vi "TestManyPublications.vi"(8 "error in (no error)":errorcluster, 11 "TestPublishRate In":refnum<class "TestManyPublications.lvclass">) -> (0 "error out":errorcluster, 3 "TestPublishRate Out":refnum<class "TestManyPublications.lvclass">)   [LabVIEW 2017, in "TestManyPublications.lvclass"]
uses:
  TestManyPublications.lvclass
  Source/Framework/IViewModel/IViewModel/IViewModel.lvclass
  C:/Git/mva-framework/Source/Framework/IViewManager/IViewManager/IViewManager.lvclass
  C:/Program Files (x86)/National Instruments/LabVIEW 2017/vi.lib/ActorFramework/Actor/Actor.lvclass
  Source/Framework/IViewable/IViewable/IViewable.lvclass
  Doubles/TestModelManyTopics/TestModelManyTopics.lvclass
  C:/Git/mva-framework/Source/Framework/IModel/IModel/IModel.lvclass
  Source/Framework/Mediator/Mediator/Mediator.lvclass
  C:/Git/mva-framework/Source/Framework/IMediator/IMediator/IMediator.lvclass
  Source/Framework/SubscriptionPolicy/ValueChangeSubscription/ValueChangeSubscription.lvclass/ValueChangeSubscription.ctl
  Source/Framework/IViewModel/IViewModel/IViewModel.lvclass/IViewModel.ctl
  Source/Framework/IViewManager/IViewManager Messages/Launch Nested Views Msg/Launch Nested Views Msg.lvclass/Launch Nested Views Msg.ctl
  Source/Framework/IViewManager/IViewManager/IViewManager.lvclass/IViewManager.ctl
  Source/Framework/Transport/QueueTransport/QueueTransport.lvclass/QueueTransport.ctl
  Source/Framework/IMediator/SubscriptionRequest/SubscriptionRequest.lvclass/SubscriptionRequest.ctl
  Source/Framework/IObserver/IObserver Messages/Subscribe Msg/Subscribe Msg.lvclass/Subscribe Msg.ctl
  <vilib>/ActorFramework/Message Enqueuer/Message Enqueuer.lvclass/Message Enqueuer.ctl
  <vilib>/ActorFramework/Stop Msg/Stop Msg.lvclass/Stop Msg.ctl
  540f04fc-0b85-431b-8f57-02b9bbd5a47e.vi
  81cf93a4-50d8-414a-8355-1077334c3962.vi
  Source/Framework/IViewModel/IViewModel/Write Startup Model-View Configuration.vi
  <vilib>/ActorFramework/Message Enqueuer/Enqueue.vi
  <vilib>/ActorFramework/Message Enqueuer/Enqueue Critical.vi
  Source/Framework/IViewManager/IViewManager Messages/Launch Nested Views Msg/Pack Launch Nested Views Msg.vi
  Source/Framework/IViewManager/IViewManager/Write Startup Launch Nested Views Msg.vi
  Source/Framework/Transport/QueueTransport/QueueTransport.lvclass
  C:/Git/mva-framework/Source/Framework/IMediator/ITransport/ITransport.lvclass
  Source/Framework/SubscriptionPolicy/ValueChangeSubscription/ValueChangeSubscription.lvclass
  C:/Git/mva-framework/Source/Framework/IMediator/ISubscriptionPolicy/ISubscriptionPolicy.lvclass
  Source/Framework/IObserver/IObserver Messages/Subscribe Msg/Subscribe Msg.lvclass
  C:/Program Files (x86)/National Instruments/LabVIEW 2017/vi.lib/ActorFramework/Message/Message.lvclass
  <vilib>/ActorFramework/Stop Msg/Stop Msg.lvclass
  <vilib>/Utility/error.llb/Error Cluster From Error Code.vi
  <vilib>/ActorFramework/Message Priority Queue/Priority Enqueue.vi
  gpm_packages/@cs/event-logger/Source/Text File Sink/Text File Sink.lvclass
  Source/Framework/IViewable/IApplicationStyle/IApplicationStyle.lvclass
  Source/Framework/IViewManager/IViewManager Messages/Launch Nested Views Msg/Launch Nested Views Msg.lvclass
  Source/Framework/IMediator/SubscriptionRequest/SubscriptionRequest.lvclass
  <vilib>/ActorFramework/Actor/Actor.lvclass
  Source/Framework/IMediator/ISubscriptionPolicy/ISubscriptionPolicy.lvclass
panel:
  out "Final Sample Transmission Time":dbl
  out "1Hz Cycle Transmission Times":dbl[](graph)
  out "Iteration":i32
  # "LV 2015 (no in-place VAT read) -- 0.53 sec typical\nLV 2017 (in-place VAT get element) -- 0.02 to 0.03 sec typical\nLV 2017 (In-place Transport) -- 0.0065 sec typical (with debug log = True)"
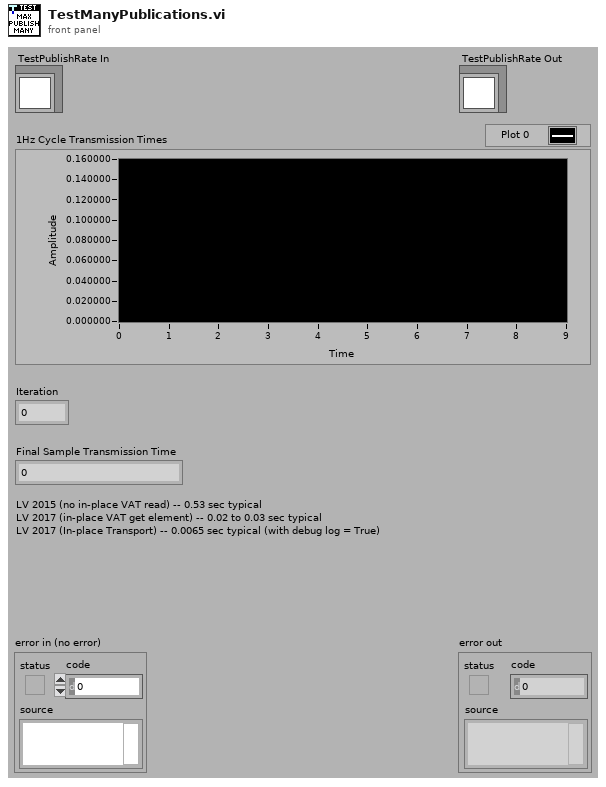
[diagram p1: front panel]
types:
  T1 = typedef "IMediator.lvlib/ISubscriptionPolicy.lvclass/ISubscriptionPolicy Reference.ctl" = refnum<data-value>
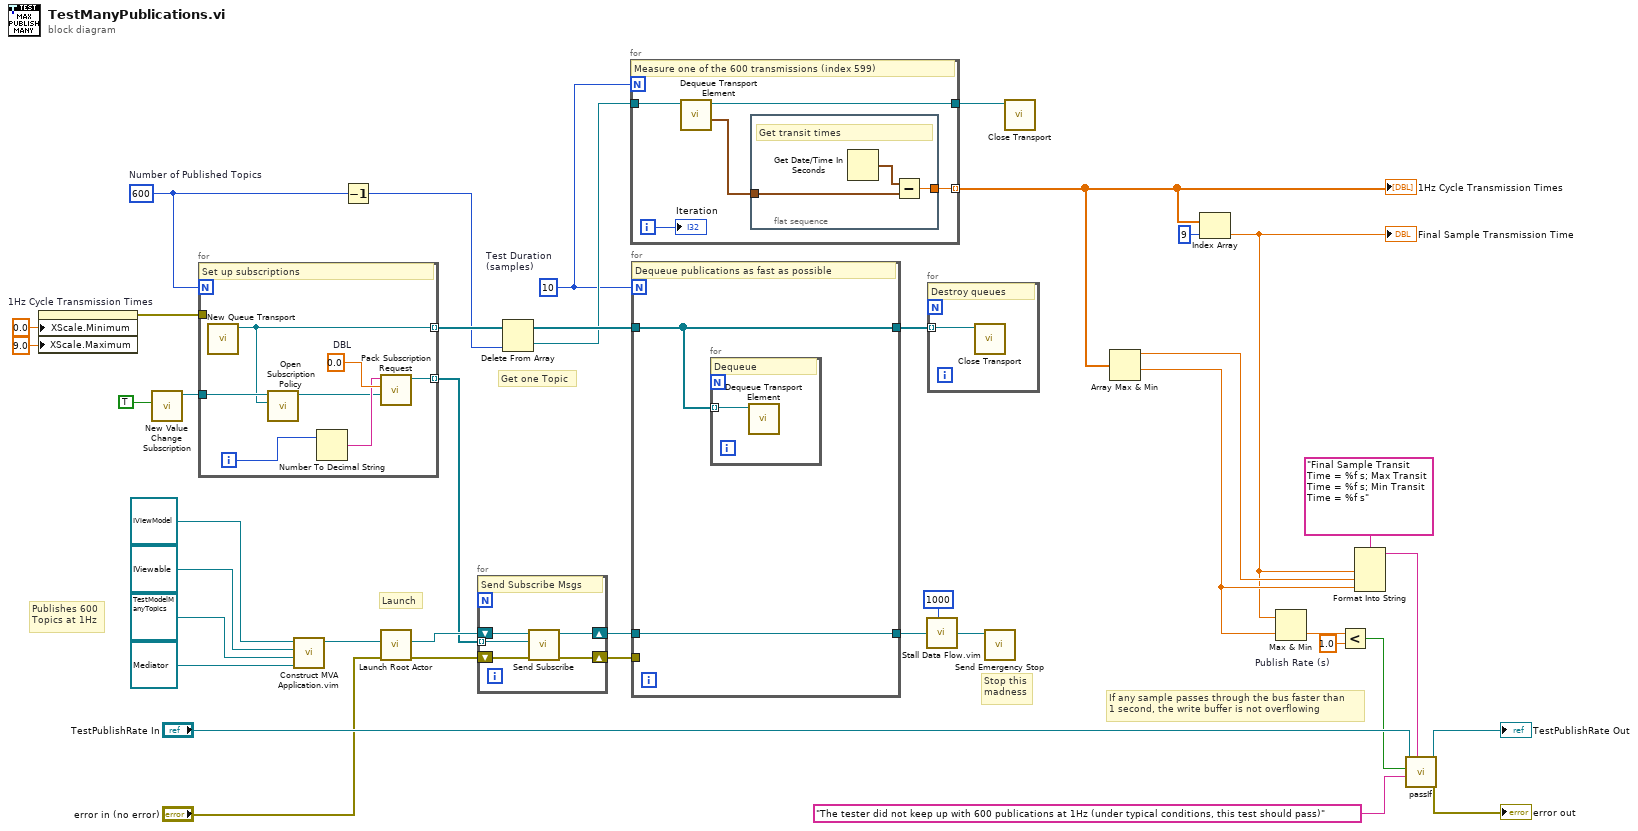
[diagram p0: block diagram]
diagram:
  w9 = 1.0  # Publish Rate (s)
  w7 = 600  # Number of Published Topics
  w17 = 10  # Test Duration (samples)
  # "Publishes 600\nTopics at 1Hz"
  # "If any sample passes through the bus faster than\n1 second, the write buffer is not overflowing"
  # "Get one Topic"
  # "Stop this\nmadness"
  # "Launch"
  n1 = property on="1Hz Cycle Transmission Times" class="WFChart (strict)"("XScale.Minimum"=0.0 ("X Scale.Range:Minimum"), "XScale.Maximum"=9.0 ("X Scale.Range:Maximum")) -> (error out=w1:errorcluster)  [unwired: 2 in, 1 out]
  n2 = call "New Value Change Subscription.vi"("Ignore Past Updates? (F)"=TRUE) -> ("ValueChangeSubscription Out"=w22:refnum<class "ValueChangeSubscription.lvclass">)  [unwired: 10 in]
  n3 = for {
    N: w7 -> [_]
    tunnel: [w48] -> w31 mode=indexing
    tunnel: w22 -> [w46]
    tunnel: [w43] -> w21 mode=indexing
    tunnel: w1 -> [_]
    i -> [w45]
    w47 = 0.0  # DBL
    # "Set up subscriptions"
    n4 = call "New Queue Transport.vi"() -> ("QueueTransport"=w43:refnum<class "QueueTransport.lvclass">)  [unwired: 10 in, 1 out]
    n5 = call "Open Subscription Policy.vi"("Transport"=w43, "SubscriptionPolicy"=w46) -> ("Subscription Policy"=w42:T1)  [unwired: 8 in, 1 out]
    n6 = Number To Decimal String(number=w45) -> (decimal integer string=w44:string)  [unwired: 1 in]
    n7 = call "Pack Subscription Request.vi"("Subscription Policy"=w42, "Type"=w47, "Datum Name"=w44) -> ("SubscriptionRequest"=w48:refnum<class "SubscriptionRequest.lvclass">)  [unwired: 8 in]
  }
  n8 = call "Construct MVA Application.vim"("Mediator Type"=refnum<class "Mediator.lvclass"> refnum ("Mediator"), "Model Type"=refnum<class "TestModelManyTopics.lvclass"> refnum ("Model"), "Startup View Configuration"=refnum<class "IViewable.lvclass"> refnum, "IViewModel In"=refnum<class "IViewModel.lvclass"> refnum) -> ("IViewModel Out"=w33:refnum<class "IViewModel.lvclass">)  [unwired: 7 in]
  n9 = Decrement(x=w7) -> (x-1=w6:i32)
  n10 = call <vilib>:"Launch Root Actor.vi"("error in (no error)"="error in (no error)", "Actor"=w33) -> ("error out"=w29:errorcluster, "Actor's Enqueuer"=w32:refnum<class "Message Enqueuer.lvclass">)  [unwired: 8 in]
  n11 = for {
    tunnel: w31 -> [w52] mode=indexing
    shift-right: [w51] -> w30
    shift-left: w32 -> [w53]
    shift-right: [w49] -> w28
    shift-left: w29 -> [w50]
    # "Send Subscribe Msgs"
    n12 = call "Send Subscribe.vi"("error in (no error)"=w50, "SubscriptionRequest"=w52, "Message Enqueuer"=w53) -> ("error out"=w49:errorcluster, "Message Enqueuer out"=w51:refnum<class "Message Enqueuer.lvclass">)  [unwired: 7 in]
  }
  n13 = Delete From Array(array=w21, index=w6) -> (deleted portion=w19:refnum<class "QueueTransport.lvclass">, array with subset deleted=w20:refnum<class "QueueTransport.lvclass">[])  [unwired: 1 in]
  n14 = for {
    N: w17 -> [_]
    tunnel: w19 -> [w58]
    tunnel: [w57] -> w18
    tunnel: [w56] -> w14 mode=indexing
    i -> [w55]
    # "Measure one of the 600 transmissions (index 599)"
    n15 = call "Dequeue Transport Element.vi"("QueueTransport in"=w58) -> ("Publication Time"=w54:timestamp, "QueueTransport out"=w57:refnum<class "QueueTransport.lvclass">)  [unwired: 7 in, 2 out]
    n16 = flat-sequence {
      tunnel: [w60] -> w56
      tunnel: w54 -> [w59]
      frame #0 {
        # "Get transit times"
        n17 = Get Date/Time In Seconds() -> (seconds since 1Jan1904=w61:timestamp)
        n18 = Subtract(x=w61, y=w59) -> (x-y=w60:dbl)
      }
    }
    "Iteration" <- w55
  }
  "1Hz Cycle Transmission Times" <- w14
  n19 = for {
    N: w17 -> [_]
    tunnel: w30 -> [w63]
    tunnel: w28 -> [_]
    tunnel: [w63] -> w27
    tunnel: [w62] -> w26
    tunnel: w20 -> [w62]
    # "Dequeue publications as fast as possible"
    n20 = for {
      tunnel: w62 -> [w64] mode=indexing
      # "Dequeue"
      n21 = call "Dequeue Transport Element.vi"("QueueTransport in"=w64) -> ()  [unwired: 7 in, 4 out]
    }
  }
  n22 = call "Stall Data Flow.vim"("value in"=w27, "milliseconds to wait"=u32 1000) -> ("value out"=w5:refnum<class "Message Enqueuer.lvclass">)  [unwired: 1 out]
  n23 = for {
    tunnel: w26 -> [w65] mode=indexing
    # "Destroy queues"
    n24 = call-dynamic "Close Transport.vi"("QueueTransport in"=w65) -> ()  [unwired: 10 in, 1 out]
  }
  n25 = call <vilib>:"Send Emergency Stop.vi"("Message Enqueuer"=w5) -> ()  [unwired: 10 in, 1 out]
  n26 = call-dynamic "Close Transport.vi"("QueueTransport in"=w18) -> ()  [unwired: 10 in, 1 out]
  n27 = Array Max & Min(array=w14) -> (max value=w13:dbl, min value=w12:dbl)  [unwired: 2 out]
  n28 = Index Array(array=w14, index=9) -> (element=w11:dbl)
  "Final Sample Transmission Time" <- w11
  n29 = Max & Min(x=w11, y=w12) -> (min(x,y)=w10:dbl)  [unwired: 1 out]
  n30 = Less?(x=w10, y=w9) -> (x < y?=w8:bool)
  n31 = Format Into String(format string="Final Sample Transit Time = %f s; Max Transit Time = %f s; Min Transit Time = %f s", w11, w13, w12) -> (resulting string=w25:string)  [unwired: 2 in, 1 out]
  n32 = call-dynamic "passIf.vi"("custom report message (\"\")"=w25, "message (\"\")"="The tester did not keep up with 600 publications at 1Hz (under typical conditions, this test should pass)" ("message (\"\")"), "pass"=w8, "TestCase in"="TestPublishRate In") -> ("error out"=→"error out":errorcluster, "TestCase out"=→"TestPublishRate Out":refnum<class "TestManyPublications.lvclass">)  [unwired: 6 in]
